vi "onKeyWrite.vi"(7 "Qualified Name":string[](array[string]), 8 "error in (no error)":errorcluster, 9 "Content":T1[](array[typedef]), 10 "Keys":string[](array[string]), 11 "ConfigManager.Text.INI in":refnum<class "ConfigManager.Text.INI.lvclass">) -> (0 "error out":errorcluster, 1 "Content out":T1[](array[typedef]), 2 "Keys out":string[](array[string]), 3 "ConfigManager.Text.INI out":refnum<class "ConfigManager.Text.INI.lvclass">, 5 "Qualified Name out":string[](array[string]))   [LabVIEW 2013, in "CfgManager.Text.lvlib" / "ConfigManager.Text.INI.lvclass"]
uses:
  ConfigManager.Text.INI.lvclass
  Manager.Text/Dictionary Payload -- cluster.ctl
  Manager.Text/ConfigManager.Text.lvclass
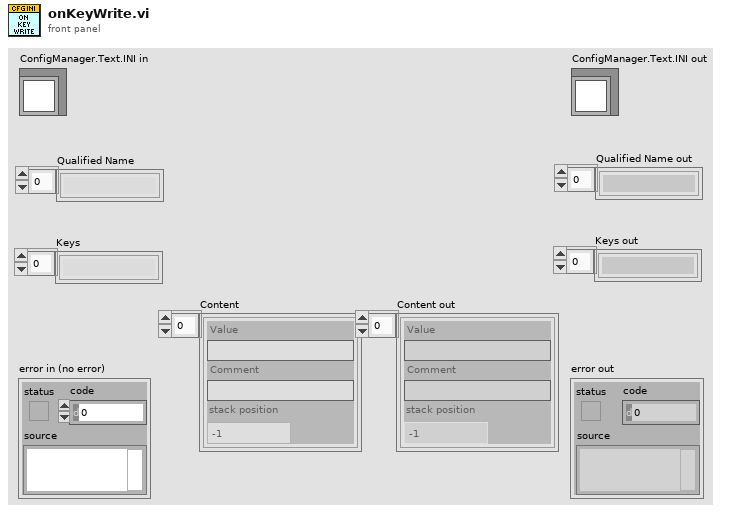
[diagram p1: front panel]
types:
  T1 = typedef "CfgManager.Text.lvlib/ConfigManager.Text.lvclass/Dictionary Payload -- cluster.ctl" = cluster{"Value":string, "Comment":string, "stack position":i32}
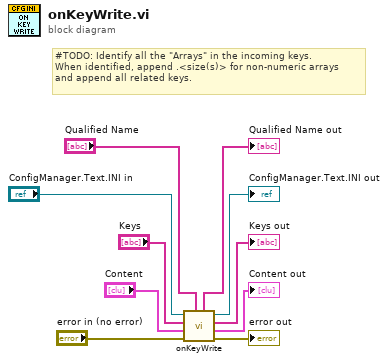
[diagram p0: block diagram]
diagram:
  # "#TODO: Identify all the \"Arrays\" in the incoming keys.\nWhen identified, append .<size(s)> for non-numeric arrays\nand append all related keys."
  n1 = call-parent "onKeyWrite.vi"("Qualified Name"="Qualified Name", "error in (no error)"="error in (no error)", "Content"="Content", "Keys"="Keys", "ConfigManager.Text in"="ConfigManager.Text.INI in") -> ("error out"=→"error out":errorcluster, "Content out"=→"Content out":T1[], "Keys out"=→"Keys out":string[], "ConfigManager.Text out"=→"ConfigManager.Text.INI out":refnum<class "ConfigManager.Text.INI.lvclass">, "Qualified Name out"=→"Qualified Name out":string[])  [unwired: 2 in]
